vi "Close.vi"(8 "error in":errorcluster, 11 "Pressure Gradient in":refnum<class "Pressure Gradient.lvclass">) -> (0 "error out":errorcluster, 3 "Pressure Gradient out":refnum<class "Pressure Gradient.lvclass">)   [LabVIEW 2023, in "Pressure Gradient.lvclass"]
uses:
  Pressure Gradient.lvclass
  Pressure Gradient.lvclass/Pressure Gradient.ctl
  Parents/Gradient/Gradient.lvclass
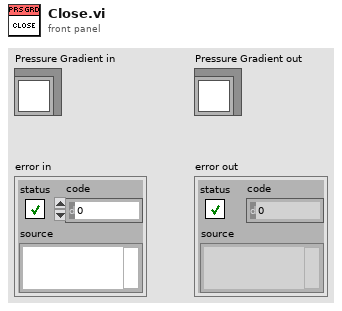
[diagram p1: front panel]
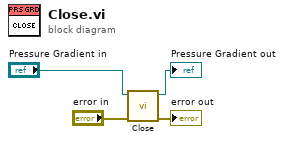
[diagram p0: block diagram]
diagram:
  n1 = call-parent "Close.vi"("error in"="error in", "Gradient in"="Pressure Gradient in") -> ("error out"=→"error out":errorcluster, "Gradient out"=→"Pressure Gradient out":refnum<class "Pressure Gradient.lvclass">)  [unwired: 8 in]
